vi "Configure Offset Compensation.vi"(8 "error in (no error)":errorcluster, 10 "Enable Offset Compensation (Enable)":bool=TRUE, 11 "VISA resource name":refnum<visa-resource-name>) -> (0 "error out":errorcluster, 3 "VISA resource name out":refnum<visa-resource-name>)   [LabVIEW 2020, in "3458A Basic Driver.lvlib"]
doc: "Configures the offset compensation functionality of the DMM."
uses:
  3458A Basic Driver.lvlib
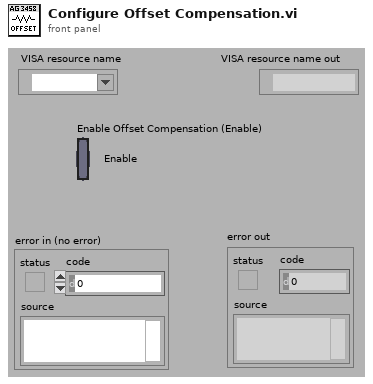
[diagram p1: front panel]
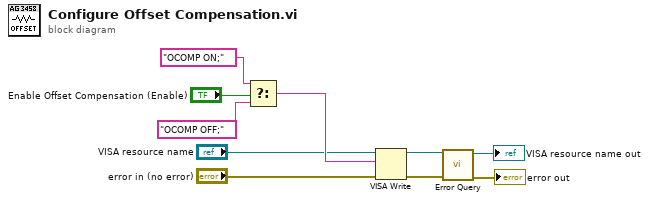
[diagram p0: block diagram]
diagram:
  n1 = Select(t="OCOMP ON;", s="Enable Offset Compensation (Enable)", f="OCOMP OFF;") -> (s? t:f=w7:string)
  n2 = VISA Write(VISA resource name="VISA resource name", write buffer=w7, error in (no error)="error in (no error)") -> (VISA resource name out=w5:refnum<visa-resource-name>, error out=w4:errorcluster)  [unwired: 1 out]
  n3 = call "Error Query.vi"("error in (no error)"=w4, "VISA resource name"=w5) -> ("error out"=→"error out":errorcluster, "VISA resource name out"=→"VISA resource name out":refnum<visa-resource-name>)  [unwired: 6 in, 2 out]
